vi "Select ROI_SLM.vi"(9 "Array In":sgl[][](array[numeric]), 10 "ROI Size":dbl, 11 "IntensityGraph in":refnum<vi>) -> (1 "ROI":sgl[][](array[numeric]))   [LabVIEW 2014]
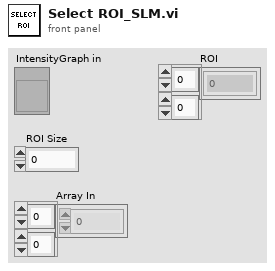
[diagram p1: front panel]
types:
  T1 = typedef "LVPointDoubleTypeDef.ctl" = cluster{"Cursor X":dbl, "Cursor Y":dbl}
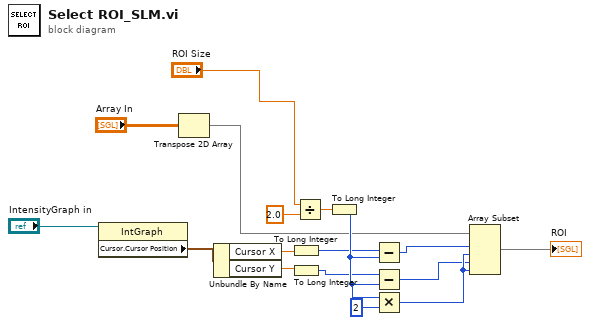
[diagram p0: block diagram]
diagram:
  n1 = property on="Property Node" class="IntGraph"(reference="IntensityGraph in") -> ("Cursor.Cursor Position"=w4:T1)  [unwired: 1 in, 2 out]
  n2 = Transpose 2D Array(2D array="Array In") -> (transposed array=w1:sgl[][])
  n3 = Unbundle By Name(w4) -> ("Cursor X"=w5:dbl, "Cursor Y"=w6:dbl)
  n4 = To Long Integer(number=w5) -> (32bit integer=w10:i32)
  n5 = To Long Integer(number=w6) -> (32bit integer=w11:i32)
  n6 = Divide(x="ROI Size", y=2.0) -> (x/y=w9:dbl)
  n7 = To Long Integer(number=w9) -> (32bit integer=w14:i32)
  n8 = Subtract(x=w10, y=w14) -> (x-y=w12:i32)
  n9 = Subtract(x=w11, y=w14) -> (x-y=w13:i32)
  n10 = Multiply(x=w14, y=2) -> (x*y=w16:i32)
  n11 = Array Subset(array=w1, index (row)=w12, length (row)=w16, index (col)=w13, length (col)=w16) -> (→"ROI":sgl[][])
